vi "DM Test.vi"() -> ()   [LabVIEW 2017]
uses:
  <vilib>/Instr/_visa.llb/VISA Configure Serial Port (Instr).vi
panel:
  in  "POWER":bool=TRUE
  out "Error Out":errorcluster
  in  "Resource Name":refnum<visa-resource-name>="ASRL1::INSTR"
  in  "Error In (no error)":errorcluster
  out "Present Wavelength":dbl format="%.2f"
  in  "Goto OK":bool
  in  "Set Wavelength":dbl=100.0 min=-100.0 max=1000.0 step=2.0 format="%.3f"
  # "nm"
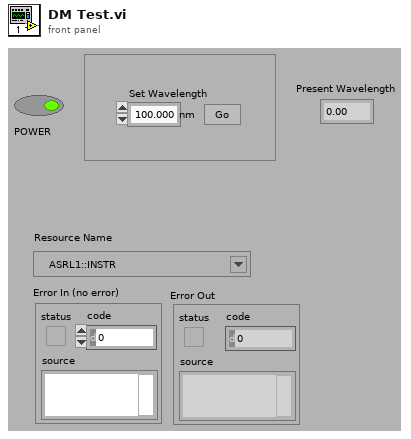
[diagram p1: front panel]
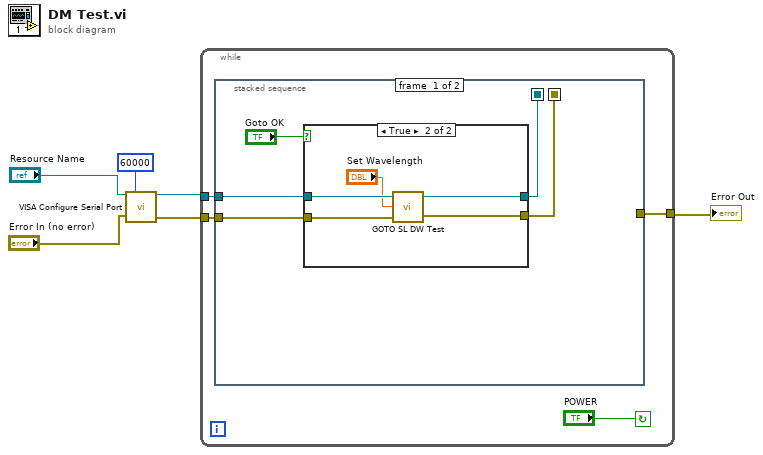
[diagram p0: block diagram]
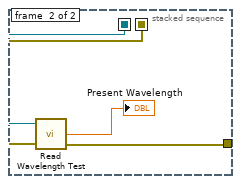
[diagram p3: hidden frame]
diagram:
  n1 = call-poly "VISA Configure Serial Port"("VISA resource name"="Resource Name", "timeout (10sec)"=60000, "error in (no error)"="Error In (no error)") -> ("VISA resource name out"=w2:refnum<visa-resource-name>, "error out"=w1:errorcluster)  [unwired: 11 in]
  n2 = while {
    tunnel: [w9] -> w3
    tunnel: w2 -> [w8]
    tunnel: w1 -> [w7]
    stop <- "POWER" continue-if-true
    n3 = stacked-sequence {
      seq-local: [w13 _] -> [_ w24]
      seq-local: [w14 _] -> [_ w25]
      tunnel: [_ w26] -> w9
      tunnel: w8 -> [w12 _]
      tunnel: w7 -> [w11 _]
      frame #0 {
        n4 = case shown="True" "Goto OK" {
          tunnel: [w16 w22] -> w13
          tunnel: [w17 w21] -> w14
          tunnel: w12 -> [w17 w20]
          tunnel: w11 -> [w16 w19]
          frame False {
          }
          frame True {
            n5 = call "GOTO SL DW Test.vi"("Error In (no error)"=w19, "Set Wavelength"="Set Wavelength", "Resource Name"=w20) -> ("Error Out"=w22:errorcluster, "Resource Name 2"=w21:refnum<visa-resource-name>)
          }
        }
      }
      frame #1 {
        n6 = call "Read Wavelength Test.vi"("Error In (no error)"=w24, "Resource Name"=w25) -> ("Error Out"=w26:errorcluster, "Wavelength"=→"Present Wavelength":dbl)  [unwired: 1 in, 1 out]
      }
    }
  }
  "Error Out" <- w3
